vi "LM Double Exponential and gradient.vi"(3 "output control":T1, 4 "data":variant, 5 "X":dbl[](array[numeric]), 6 "a":dbl[](array[numeric])) -> (0 "error out":errorcluster, 1 "f'(X,a)":dbl[][](array[numeric]), 2 "f(X,a)":dbl[](array[numeric]))   [LabVIEW 2021, in "Fits.lvlib"]
doc: "This template is the starting point for creating a model function to be passed to the Nonlinear Curve Fit.vi."
uses:
  Fits.lvlib
  <vilib>/gmath/NumericalOptimization/LM_output select.ctl
  <vilib>/gmath/NI_Gmath.lvlib
panel:
  # "Parameters:\n\nA1, t1\nA2, t2\nB"
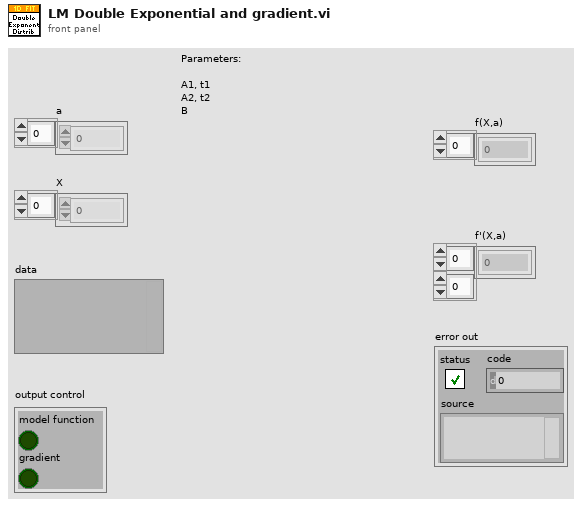
[diagram p1: front panel]
types:
  T1 = typedef "NI_Gmath.lvlib/LM_output select.ctl" = cluster{"model function":bool, "gradient":bool}
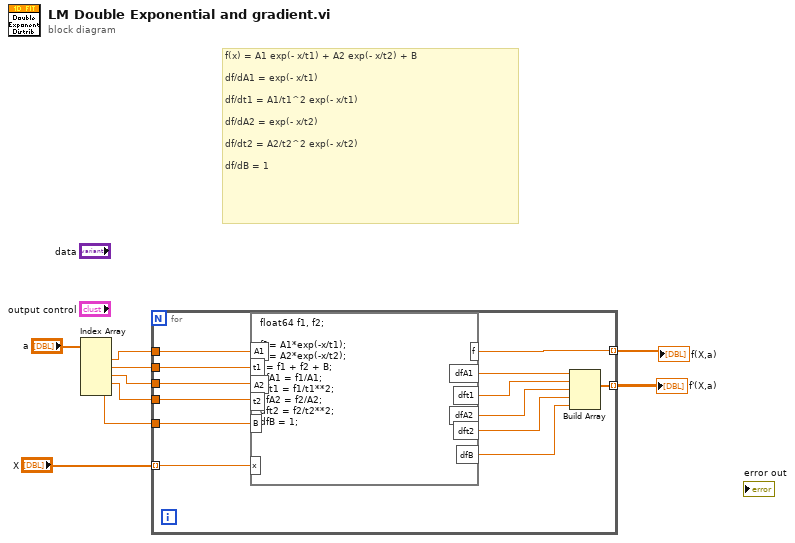
[diagram p0: block diagram]
diagram:
  # "f(x) = A1 exp(- x/t1) + A2 exp(- x/t2) + B\n \ndf/dA1 = exp(- x/t1)     \n\ndf/dt1 = A1/t1^2 exp(- x/t1) \n\ndf/dA2 = exp(- x/t2)     \n\ndf/dt2 = A2/t2^2 exp(- x/t2) \n\ndf/dB = 1"
  n1 = Index Array(array="a") -> (element #1=w8:dbl, element #2=w7:dbl, element #3=w6:dbl, element #4=w5:dbl, element #5=w1:dbl)  [unwired: 5 in]
  n2 = for {
    tunnel: w8 -> [w22]
    tunnel: w7 -> [w21]
    tunnel: w6 -> [w15]
    tunnel: w5 -> [w14]
    tunnel: "X" -> [w20] mode=indexing
    tunnel: [w18] -> w3 mode=indexing
    tunnel: [w16] -> w2 mode=indexing
    tunnel: w1 -> [w11]
    n3 = formula code="float64 f1, f2;\n\nf1= A1*exp(-x/t1);\nf2= A2*exp(-x/t2);\nf = f1 + f2 + B;\ndfA1 = f1/A1;\ndft1 = f1/t1**2;\ndfA2 = f2/A2;\ndft2 = f2/t2**2;\ndfB = 1;"("A1"=w22, "t1"=w21, "A2"=w15, "x"=w20, "t2"=w14, "B"=w11) -> ("f"=w18:dbl, "dfA1"=w19:dbl, "dft1"=w17:dbl, "dfA2"=w13:dbl, "dft2"=w12:dbl, "dfB"=w10:dbl)
    n4 = Build Array(w19, w17, w13, w12, w10) -> (w16:dbl[])
  }
  "f(X,a)" <- w3
  "f'(X,a)" <- w2
